vi "Execute.vi"(8 "error in":errorcluster, 11 "Std MSG STEP in":refnum<class "String STEP.lvclass">) -> (0 "error out":errorcluster, 1 "Next Step?":bool, 2 "MSG":string, 3 "Std MSG STEP out":refnum<class "String STEP.lvclass">)   [LabVIEW 2014, in "String STEP.lvclass"]
doc: "This implementation of the STEP class is used to output simple string messages."
uses:
  String STEP.lvclass
  String STEP.lvclass/String STEP.ctl
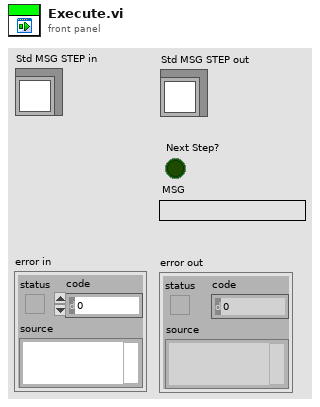
[diagram p1: front panel]
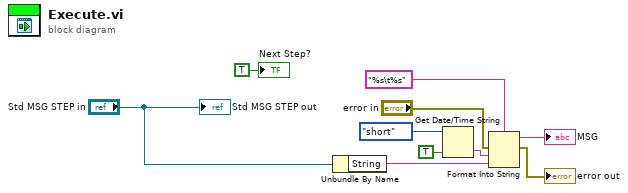
[diagram p0: block diagram]
diagram:
  n1 = Unbundle By Name("Std MSG STEP in") -> ("String"=w4:string)
  n2 = Get Date/Time String(date format (0)=enum16{"short", "long", "abbreviated"}."short", want seconds? (F)=TRUE) -> (time string=w7:string)  [unwired: 1 in, 1 out]
  n3 = Format Into String(format string="%s\t%s", error in="error in", w7, w4) -> (resulting string=→"MSG":string, error out=→"error out":errorcluster)  [unwired: 1 in]
  "Std MSG STEP out" <- "Std MSG STEP in"
  "Next Step?" <- TRUE ("Next Step?")
